vi "Write enemy_ball_possesion.vi"(8 "error in (no error)":errorcluster, 10 "enemy_ball_possesion":bool, 11 "Events in":refnum<class "Events.lvclass">) -> (0 "error out":errorcluster, 3 "Events out":refnum<class "Events.lvclass">)   [LabVIEW 2023, in "Events.lvclass"]
uses:
  Events.lvclass
  Events.lvclass/Events.ctl
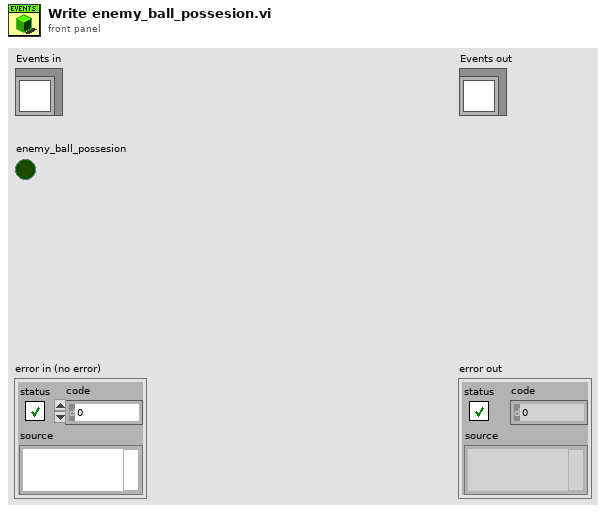
[diagram p1: front panel]
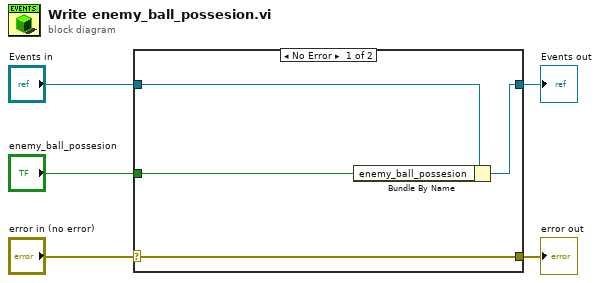
[diagram p0: block diagram]
diagram:
  n1 = case shown="No Error" "error in (no error)" {
    selector: "error in (no error)" -> [w9 w10]
    tunnel: [w9 w10] -> w4
    tunnel: [w7 w11] -> w2
    tunnel: "Events in" -> [w8 w11]
    tunnel: "enemy_ball_possesion" -> [w6 _]
    frame No Error {
      n2 = Bundle By Name(cluster=w8, "enemy_ball_possesion"=w6) -> (w7:refnum<class "Events.lvclass">)
    }
    frame Error {
    }
  }
  "error out" <- w4
  "Events out" <- w2
